vi "xyCourdinte.vi"(2 "Y":dbl, 3 "X":dbl, 4 "speed":i32(knob) scale=0.0..5.0, 5 "angle":i32) -> (0 "yResult":dbl format="%#_4f", 1 "xResult":dbl format="%#_6f")   [LabVIEW 2013]
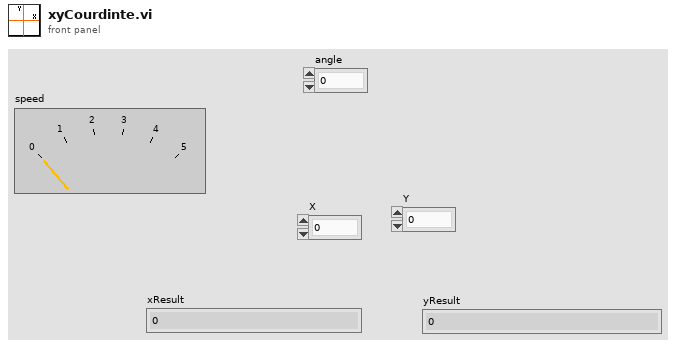
[diagram p1: front panel]
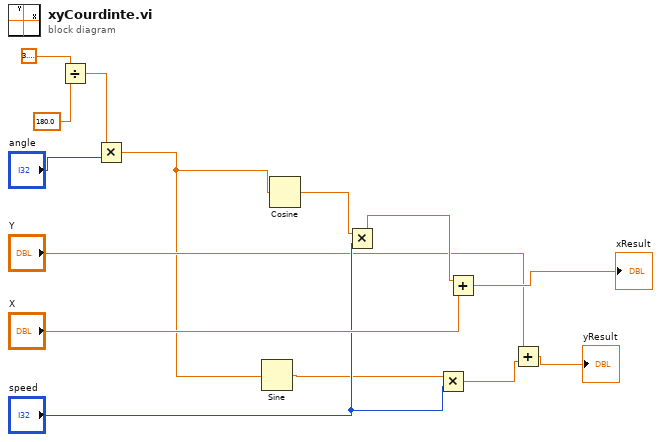
[diagram p0: block diagram]
diagram:
  n1 = Divide(x=3.141592653589793, y=180.0) -> (x/y=w5:dbl)
  n2 = Multiply(x=w5, y="angle") -> (x*y=w4:dbl)
  n3 = Sine(x=w4) -> (sin(x)=w2:dbl)
  n4 = Cosine(x=w4) -> (cos(x)=w3:dbl)
  n5 = Multiply(x=w3, y="speed") -> (x*y=w13:dbl)
  n6 = Multiply(x=w2, y="speed") -> (x*y=w10:dbl)
  n7 = Add(x=w13, y="X") -> (x+y=→"xResult":dbl)
  n8 = Add(x="Y", y=w10) -> (x+y=→"yResult":dbl)
